vi "PingPong.vi"() -> ()   [LabVIEW 2023, in "CTI-Visa-Scratchpad.lvlib"]
uses:
  CTI-Visa-Scratchpad.lvlib
  CTI-Visa/Digital Direction.ctl
  CTI-Visa/Digital Pull Direction.ctl
  CTI-Visa/CTI-Visa.lvlib
panel:
  out "error out":errorcluster
  in  "Stop":bool
  in  "VISA resource":refnum<visa-resource-name>
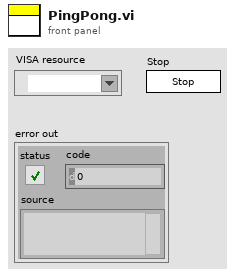
[diagram p1: front panel]
types:
  T1 = typedef "CTI-Visa.lvlib/Digital Direction.ctl" = enum16{"In", "Out"}
  T2 = typedef "CTI-Visa.lvlib/Digital Pull Direction.ctl" = enum16{"None", "Up", "Down", "Both"}
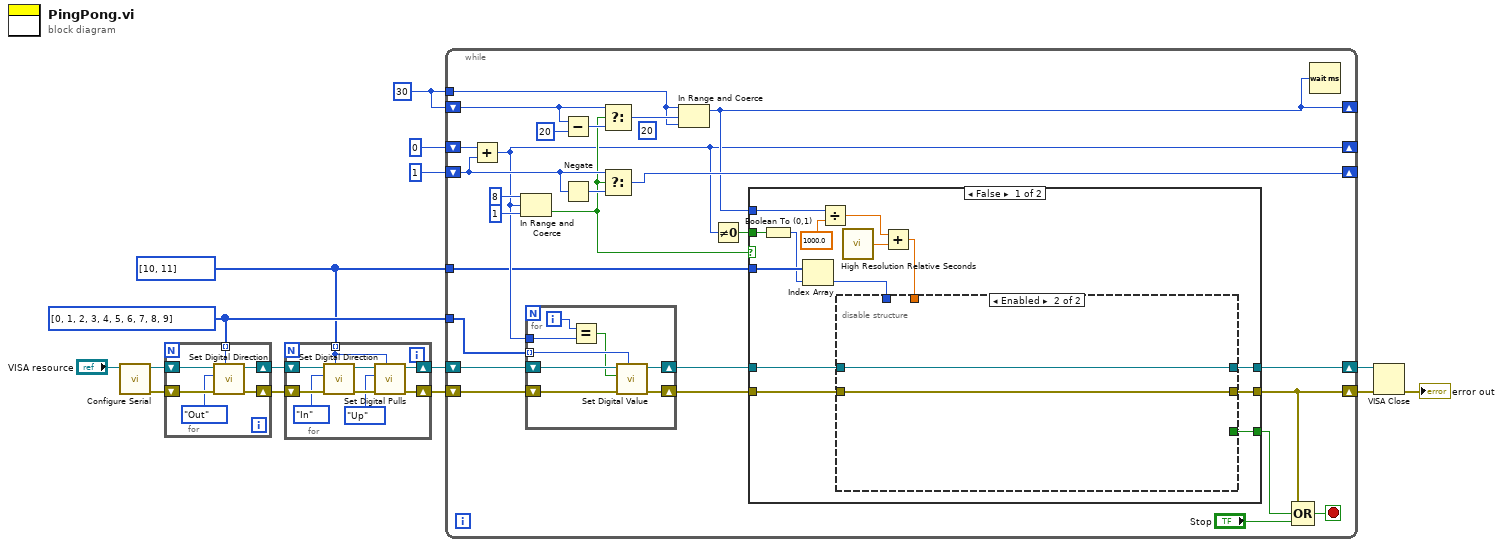
[diagram p0: block diagram]
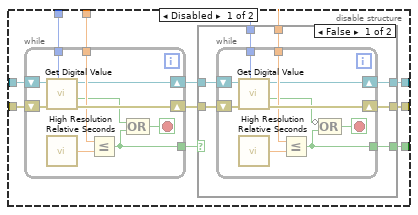
[diagram p2: hidden frame]
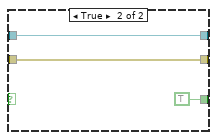
[diagram p3: hidden frame]
diagram:
  w2 = 30
  w1 = i32[] [10, 11]
  w6 = i32[] [0, 1, 2, 3, 4, 5, 6, 7, 8, 9]
  n1 = call "Configure Serial.vi"("VISA resource name in"="VISA resource") -> ("error out"=w15:errorcluster, "VISA resource name"=w13:refnum<visa-resource-name>)  [unwired: 9 in]
  n2 = for {
    shift-right: [w17] -> w12
    shift-left: w13 -> [w20]
    shift-right: [w16] -> w11
    shift-left: w15 -> [w21]
    tunnel: w6 -> [w18] mode=indexing
    n3 = call "Set Digital Direction.vi"("GPIO"=w18, "error in (no error)"=w21, "Direction"=Digital_Direction."Out", "VISA resource name in"=w20) -> ("error out"=w16:errorcluster, "VISA resource name"=w17:refnum<visa-resource-name>)  [unwired: 6 in]
  }
  n4 = for {
    shift-right: [w22] -> w9
    shift-left: w12 -> [w29]
    shift-right: [w23] -> w10
    shift-left: w11 -> [w30]
    tunnel: w1 -> [w25] mode=indexing
    n5 = call "Set Digital Direction.vi"("GPIO"=w25, "error in (no error)"=w30, "Direction"=Digital_Direction."In", "VISA resource name in"=w29) -> ("error out"=w26:errorcluster, "VISA resource name"=w27:refnum<visa-resource-name>)  [unwired: 6 in]
    n6 = call "Set Digital Pulls.vi"("GPIO"=w25, "error in (no error)"=w26, "Pull"=Digital_Pull_Direction."Up", "VISA resource name in"=w27) -> ("error out"=w23:errorcluster, "VISA resource name"=w22:refnum<visa-resource-name>)  [unwired: 6 in]
  }
  n7 = while {
    shift-right: [w34] -> w5
    shift-left: w10 -> [w48]
    shift-right: [w33] -> w4
    shift-left: w9 -> [w49]
    shift-right: [w37] -> _
    shift-left: 0 -> [w56]
    shift-right: [w51] -> _
    shift-left: 1 -> [w52]
    shift-right: [w39] -> _
    shift-left: w2 -> [w43]
    tunnel: w6 -> [w50]
    tunnel: w2 -> [w31]
    tunnel: w1 -> [w35]
    stop <- w46 stop-if-true
    (unwired) 20 ("lower limit")
    n8 = Add(x=w56, y=w52) -> (x+y=w37:i32)
    n9 = In Range and Coerce(upper limit=8, x=w37, lower limit=1) -> (In Range?=w38:bool)  [unwired: 1 out]
    n10 = for {
      tunnel: w50 -> [w120] mode=indexing
      shift-right: [w115] -> w41
      shift-left: w49 -> [w122]
      shift-right: [w116] -> w40
      shift-left: w48 -> [w121]
      tunnel: w37 -> [w119]
      i -> [w118]
      n11 = Equal?(x=w118, y=w119) -> (x = y?=w117:bool)
      n12 = call "Set Digital Value.vi"("GPIO"=w120, "error in (no error)"=w121, "Value"=w117, "VISA resource name in"=w122) -> ("error out"=w116:errorcluster, "VISA resource name"=w115:refnum<visa-resource-name>)  [unwired: 6 in]
    }
    n13 = Subtract(x=w43, y=20) -> (x-y=w44:i32)
    n14 = Negate(x=w52) -> (-x=w53:i32)
    n15 = Select(t=w43, s=w38, f=w44) -> (s? t:f=w42:i32)
    n16 = Select(t=w52, s=w38, f=w53) -> (s? t:f=w51:i32)
    n17 = In Range and Coerce(upper limit=w31, x=w42, lower limit=w31) -> (coerced(x)=w39:i32)  [unwired: 1 out]
    n18 = Not Equal To 0?(x=w37) -> (x != 0?=w36:bool)
    n19 = case shown="False" w38 {
      tunnel: w41 -> [w62 w113]
      tunnel: w40 -> [w63 w114]
      tunnel: w39 -> [w67 _]
      tunnel: w36 -> [w70 _]
      tunnel: w35 -> [w69 _]
      tunnel: [w59 w114] -> w34
      tunnel: [w58 w113] -> w33
      tunnel: [w57 _] -> w32
      frame False {
        n20 = Boolean To (0,1)(Boolean=w70) -> (0, 1=w68:i16)
        n21 = Index Array(array=w69, index=w68) -> (element=w60:i32)
        n22 = Divide(x=w67, y=1000.0) -> (x/y=w64:dbl)
        n23 = call <vilib>:"High Resolution Relative Seconds.vi"() -> ("relative seconds"=w65:dbl)
        n24 = Add(x=w64, y=w65) -> (x+y=w61:dbl)
        n25 = disable-structure shown="Enabled" {
          disable-tunnel: w63 -> [w80 w111]
          disable-tunnel: w62 -> [w79 w112]
          disable-tunnel: w61 -> [w78 _]
          disable-tunnel: w60 -> [w77 _]
          disable-tunnel: [w73 w111] -> w59
          disable-tunnel: [w72 w112] -> w58
          disable-tunnel: [w71 _] -> w57
          frame Disabled {
            n26 = while {
              shift-right: [w90] -> w75
              shift-left: w80 -> [w88]
              shift-right: [w84] -> w76
              shift-left: w79 -> [w89]
              tunnel: w77 -> [w87]
              tunnel: w78 -> [w85]
              tunnel: [w81] -> w74
              stop <- w82 stop-if-true
              n27 = call "Get Digital Value.vi"("GPIO"=w87, "error in (no error)"=w88, "VISA resource name in"=w89) -> ("error out"=w90:errorcluster, "Value"=w83:bool, "VISA resource name"=w84:refnum<visa-resource-name>)  [unwired: 6 in]
              n28 = call <vilib>:"High Resolution Relative Seconds.vi"() -> ("relative seconds"=w86:dbl)
              n29 = Less Or Equal?(x=w85, y=w86) -> (x <= y?=w81:bool)
              n30 = Compound Arithmetic op=OR(w83, w81) -> (w82:bool)
            }
            n31 = case shown="False" w74 {
              tunnel: w78 -> [w97 _]
              tunnel: w77 -> [w96 _]
              tunnel: w76 -> [w95 w110]
              tunnel: w75 -> [w94 w109]
              tunnel: [w93 w110] -> w72
              tunnel: [w92 w109] -> w73
              tunnel: [w91 TRUE] -> w71
              frame False {
                n32 = while {
                  shift-right: [w107] -> w92
                  shift-left: w94 -> [w105]
                  shift-right: [w101] -> w93
                  shift-left: w95 -> [w106]
                  tunnel: w96 -> [w104]
                  tunnel: w97 -> [w102]
                  tunnel: [w98] -> w91
                  stop <- w99 stop-if-true
                  n33 = call "Get Digital Value.vi"("GPIO"=w104, "error in (no error)"=w105, "VISA resource name in"=w106) -> ("error out"=w107:errorcluster, "Value"=w100:bool, "VISA resource name"=w101:refnum<visa-resource-name>)  [unwired: 6 in]
                  n34 = call <vilib>:"High Resolution Relative Seconds.vi"() -> ("relative seconds"=w103:dbl)
                  n35 = Less Or Equal?(x=w102, y=w103) -> (x <= y?=w98:bool)
                  n36 = Compound Arithmetic op=OR(invert w100, w98) -> (w99:bool)
                }
              }
              frame True {
              }
            }
          }
          frame Enabled {
          }
        }
      }
      frame True {
      }
    }
    n37 = Compound Arithmetic op=OR(w34, w32, "Stop") -> (w46:bool)
    n38 = Wait (ms)(milliseconds to wait=w39) -> ()  [unwired: 1 out]
  }
  n39 = VISA Close(VISA resource name=w4, error in (no error)=w5) -> (error out=→"error out":errorcluster)
